vi "test poly test.vi"(10 "x":dbl) -> (2 "x+1":dbl)   [LabVIEW 2010]
uses:
  poly test (double).vi
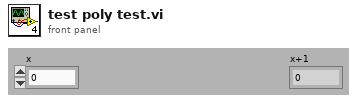
[diagram p1: front panel]
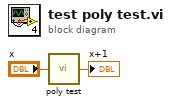
[diagram p0: block diagram]
diagram:
  n1 = call-poly "poly test.vi"("x"="x") -> ("x+1"=→"x+1":dbl)
